vi "Maximum Corr coeff.vi"() -> (5 "Plug in titles":string[](array[string]), 7 "Plug in values":string[](array[string]))   [LabVIEW 2012]
uses:
  <vilib>/Analysis/3filter.llb/Filter Passband Type.ctl
  Globals/Meas_global.vi
  <vilib>/Analysis/3filter.llb/Zero Phase Filter (Cascade, DBL).vi
  <vilib>/Analysis/NI_AALBase.lvlib
panel:
  in  "Wind turbine location":dbl=10000.0
  out "XY Graph 3":cluster{"Time (ms)":dbl[], "Eng Values":dbl[]}[](graph)
  out "?":i32
  in  "Invert values?":bool
  in  "Filter 2nd Instrument data?":bool
  in  "Freq Cutoff Inst 2":dbl=100.0
  in  "Freq Cutoff Inst 1":dbl=100.0
  in  "Filter 1st Instrument Data?":bool
  out "Time for max corr coeff":dbl
  out "Max corr coeff":dbl
  in  "Start point":dbl
  in  "Time step":dbl
  in  "Input own variables?":bool=TRUE
  out "Start point":dbl
  out "XY Graph 2":cluster{dbl[], dbl[]}(graph)
  out "Time step":dbl
  in  "Number of estimates":i32
  out "XY Graph":cluster{"Time (ms)":dbl[], "Eng Values":dbl[]}[](graph)
  in  "Instrumnt 2":i32=1
  in  "Instrument 1":i32
  # "Time lag"
  # "Correlation"
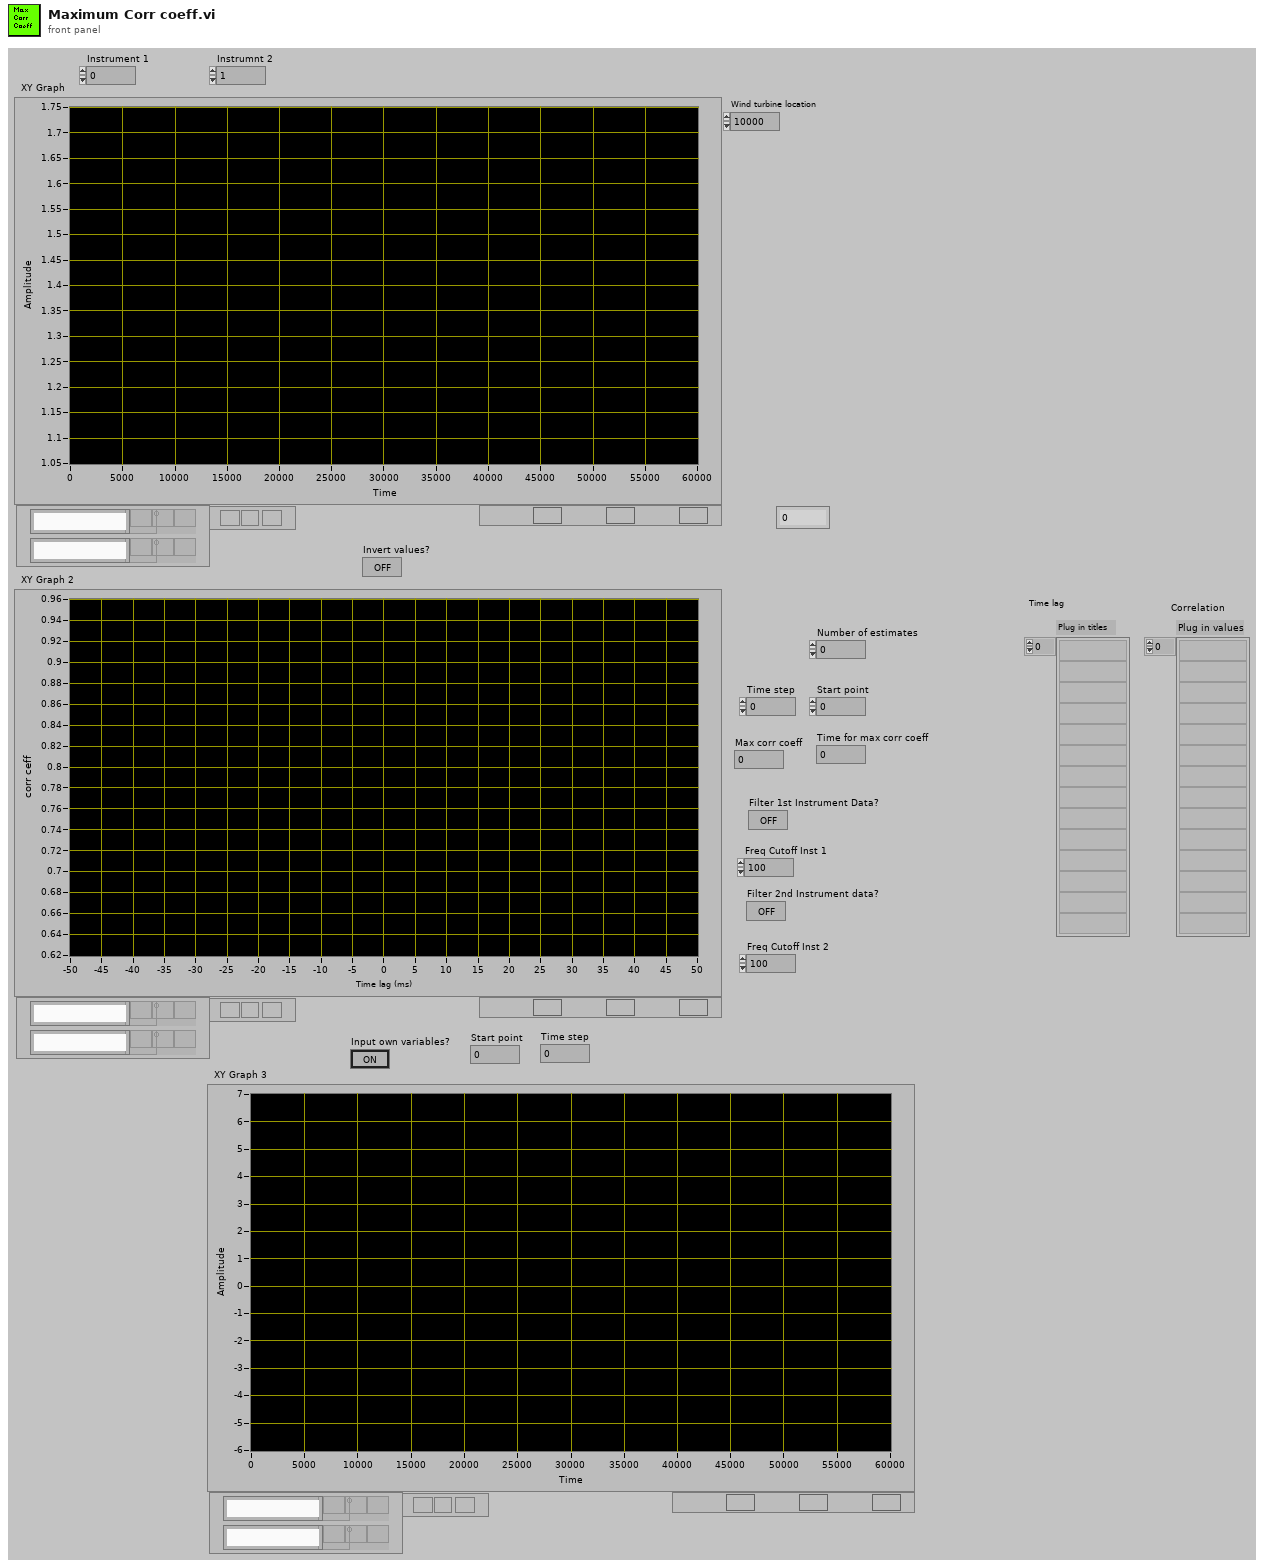
[diagram p1: front panel]
types:
  T1 = cluster{"Weighting":dbl[], "Time (ms)":dbl[], "Voltage":dbl[], "Eng Values":dbl[]}[]
  T2 = cluster{"Weighting":dbl[], "Time (ms)":dbl[], "Voltage":dbl[], "Eng Values":dbl[]}
  T3 = typedef "Analysis_info_cluster.ctl" = cluster{"Colour":u32, "Inst type":T4, "Inst name":string, "Symbol":string, "Code name":string, "Extra Info":string, "Inst Array":T5, "Extra Titles":string[], "Extra Values":string[], "U":dbl, "u^2":dbl, "u^3":dbl, "u^4":dbl, "Skew_u":dbl, "Kurt_u":dbl, "Sd Error in Mean":dbl, "% u'/U":dbl, "X":dbl, "Y":dbl, "Z":dbl, "Timescale integral to 25%":dbl, "Sd Error in Variance":dbl, "Calib File":path, "Calib Constants":dbl[], "Output Position":bool, "Full Stats":bool, "Av Sampling Rate":dbl, "Av No of Samples":dbl, "Total Meas Time (s)":dbl, "ADAM Ch Name":string}
  T4 = typedef "Inst_type.ctl" = enum16{"Propeller anemometer", "Raw voltage", "Pressure Transducer", "Pitot-static tube", "Preston tube", "Hot wire", "Cross wire 1", "Cross wire 2", "Generic Linear", "Generic Polynomial", "Generic BackPoly", "Fast FID", "Thermocouple", "Cold wire", "Pulsed Wire", "LDA Vel", "LDA Tran time", "LDA Arr time"}
  T5 = typedef "Instrument_Array.ctl" = enum16{"PWA", "LDA", "Analogue"}
  T6 = typedef "NI_AALBase.lvlib/Filter Passband Type.ctl" = enum32{"Lowpass", "Highpass", "Bandpass", "Bandstop"}
  T7 = cluster{"filter structure":enum32{"IIR 2nd Order", "IIR 4th Order"}, "Reverse Coefficients":dbl[], "Forward Coefficients":dbl[]}
  T8 = typedef "Correlation_cluster1.ctl" = cluster{"U inst":string, "uw":dbl, "u^2w":dbl, "uw^2":dbl, "uw/u'w'":dbl, "W inst":string, "uw^3":dbl, "u^3w":dbl, "u^2w^2":dbl, "Index U":i32, "Index W":i32}
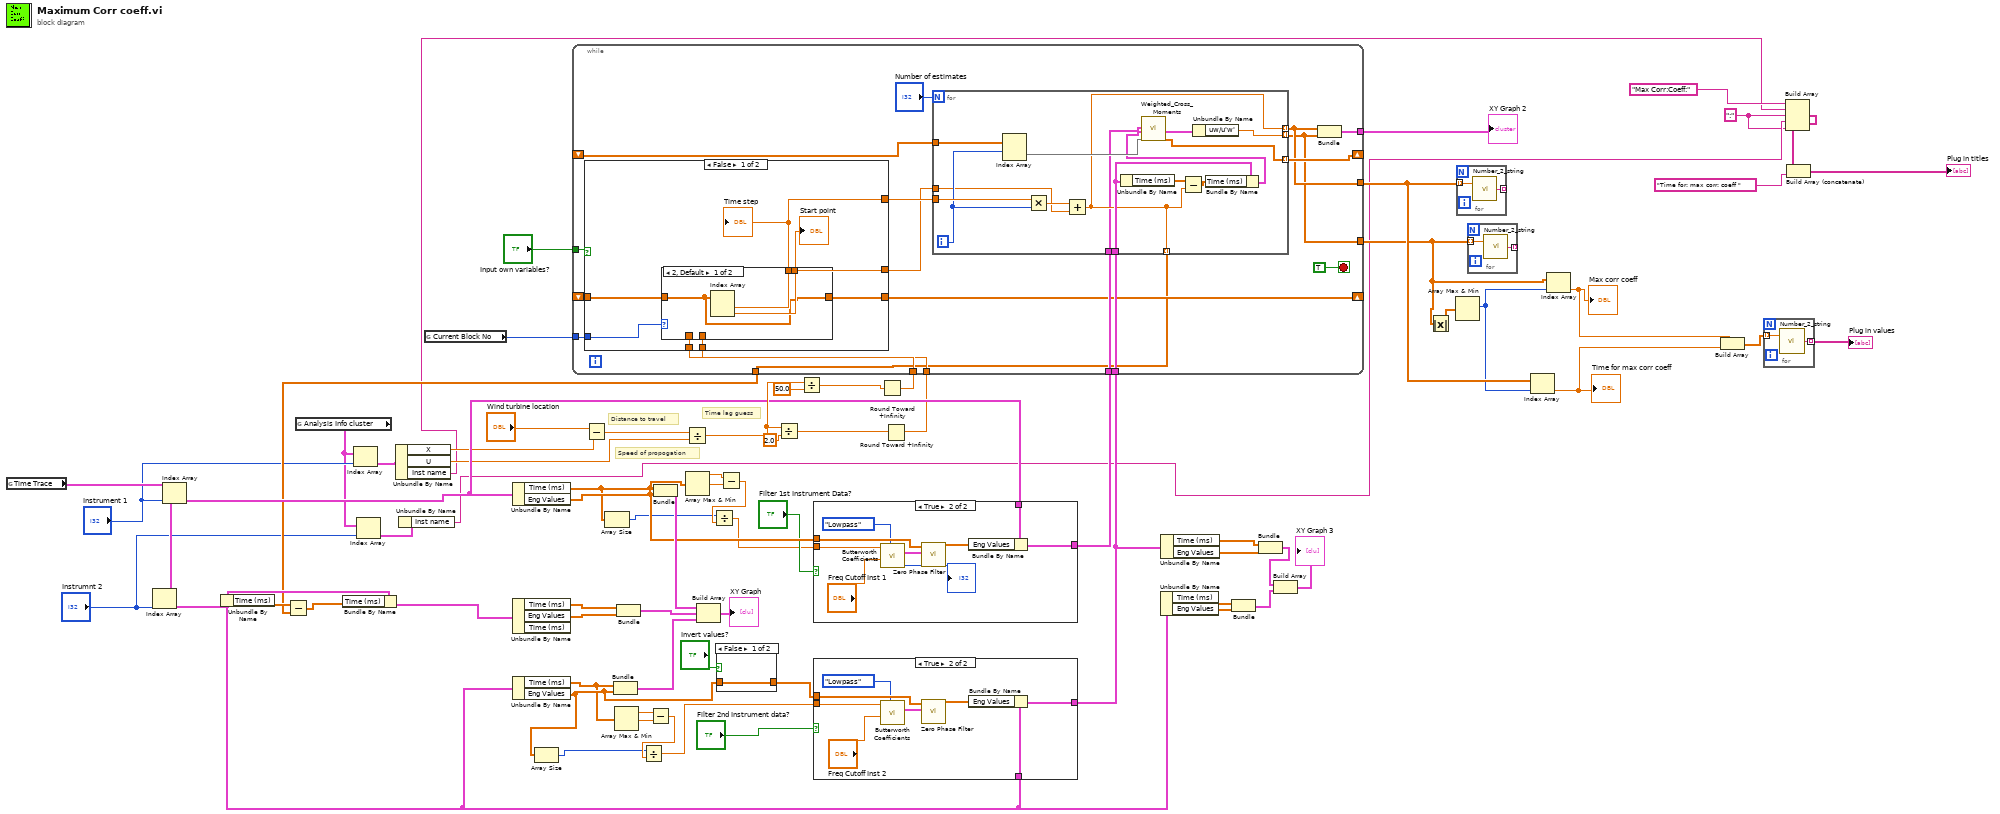
[diagram p0: block diagram]
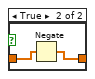
[diagram p2: hidden frame]
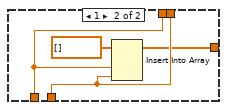
[diagram p5: hidden frame]
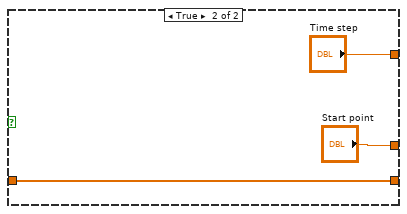
[diagram p6: hidden frame]
diagram:
  w1 = ":" ("element")
  # "Speed of propogation"
  # "Distance to travel"
  # "Time lag guess"
  n1 = global read "Meas_global.vi" "Time Trace"() -> (w68:T1)
  n2 = Index Array(array=w68, index="Instrumnt 2") -> (element=w43:T2)
  n3 = Index Array(array=w68, index="Instrument 1") -> (element=w45:T2)
  n4 = Unbundle By Name(w43) -> ("Time (ms)"=w67:dbl[])
  n5 = global read "Meas_global.vi" "Analysis Info cluster"() -> (w8:T3[])
  n6 = Index Array(array=w8, index="Instrument 1") -> (element=w22:T3)
  n7 = Index Array(array=w8, index="Instrumnt 2") -> (element=w9:T3)
  n8 = Unbundle By Name(w22) -> ("X"=w21:dbl, "U"=w20:dbl, "Inst name"=w5:string)
  n9 = Unbundle By Name(w9) -> ("Inst name"=w2:string)
  n10 = global read "Meas_global.vi" "Current Block No"() -> (w61:i32)
  n11 = Unbundle By Name(w45) -> ("Time (ms)"=w37:dbl[], "Eng Values"=w58:dbl[])
  n12 = Unbundle By Name(w43) -> ("Time (ms)"=w25:dbl[], "Eng Values"=w26:dbl[])
  n13 = Array Size(array=w26) -> (size(s)=w27:i32)
  n14 = Subtract(x="Wind turbine location", y=w21) -> (x-y=w19:dbl)
  n15 = Array Size(array=w37) -> (size(s)=w33:i32)
  n16 = Bundle("Time (ms)"=w25, "Eng Values"=w26) -> (w72:cluster{"Time (ms)":dbl[], "Eng Values":dbl[]})  [unwired: 1 in]
  n17 = Array Max & Min(array=w25) -> (max value=w29:dbl, min value=w30:dbl)  [unwired: 2 out]
  n18 = Subtract(x=w29, y=w30) -> (x-y=w28:dbl)
  n19 = Divide(x=w27, y=w28) -> (x/y=w31:dbl)
  n20 = Bundle("Time (ms)"=w37, "Eng Values"=w58) -> (w73:cluster{"Time (ms)":dbl[], "Eng Values":dbl[]})  [unwired: 1 in]
  n21 = Divide(x=w19, y=w20) -> (x/y=w63:dbl)
  n22 = Array Max & Min(array=w37) -> (max value=w36:dbl, min value=w35:dbl)  [unwired: 2 out]
  n23 = case shown="False" "Invert values?" {
    tunnel: w26 -> [w75 w76]
    tunnel: [w75 w77] -> w47
    frame False {
    }
    frame True {
      n24 = Negate(x=w76) -> (-x=w77:dbl[])
    }
  }
  n25 = Subtract(x=w36, y=w35) -> (x-y=w34:dbl)
  n26 = Divide(x=w33, y=w34) -> (x/y=w32:dbl)
  n27 = Divide(x=w63, y=2.0) -> (x/y=w17:dbl)
  n28 = Divide(x=w63, y=50.0) -> (x/y=w16:dbl)
  n29 = case shown="True" "Filter 1st Instrument Data?" {
    tunnel: w58 -> [_ w86]
    tunnel: w32 -> [_ w85]
    tunnel: w45 -> [w78 w83]
    tunnel: [w78 w82] -> w57
    frame False {
    }
    frame True {
      n30 = call <vilib>:"Butterworth Coefficients.vi"("filter type"=Filter_Passband_Type."Lowpass", "low cutoff freq: fl"="Freq Cutoff Inst 1", "sampling freq: fs"=w85) -> ("error"=→"?":i32, "IIR Filter Cluster"=w87:T7)  [unwired: 7 in]
      n31 = call-poly <vilib>:"Zero Phase Filter.vi"("IIR Filter Cluster"=w87, "X"=w86) -> ("Filtered X"=w84:dbl[])  [unwired: 8 in, 1 out]
      n32 = Bundle By Name(cluster=w83, "Eng Values"=w84) -> (w82:T2)
    }
  }
  n33 = case shown="True" "Filter 2nd Instrument data?" {
    tunnel: w47 -> [_ w95]
    tunnel: w31 -> [_ w94]
    tunnel: [w88 w92] -> w44
    tunnel: w43 -> [w88 w90]
    frame False {
    }
    frame True {
      n34 = call <vilib>:"Butterworth Coefficients.vi"("filter type"=Filter_Passband_Type."Lowpass", "low cutoff freq: fl"="Freq Cutoff Inst 2", "sampling freq: fs"=w94) -> ("IIR Filter Cluster"=w96:T7)  [unwired: 7 in, 1 out]
      n35 = call-poly <vilib>:"Zero Phase Filter.vi"("IIR Filter Cluster"=w96, "X"=w95) -> ("Filtered X"=w93:dbl[])  [unwired: 8 in, 1 out]
      n36 = Bundle By Name(cluster=w90, "Eng Values"=w93) -> (w92:T2)
    }
  }
  n37 = Round Toward +Infinity(x=w16) -> (ceil(x): smallest int >= x=w15:dbl)
  n38 = Round Toward +Infinity(x=w17) -> (ceil(x): smallest int >= x=w18:dbl)
  n39 = while {
    tunnel: w57 -> [w114]
    tunnel: w44 -> [w113]
    shift-right: [w111] -> _
    shift-left: _ -> [w110]
    tunnel: [w109] -> w65
    tunnel: [w107] -> w59
    tunnel: [w100] -> w38
    tunnel: w15 -> [w105]
    tunnel: w61 -> [w106]
    tunnel: w18 -> [w104]
    shift-right: [w103] -> _
    shift-left: _ -> [w102]
    tunnel: "Input own variables?" -> [w99]
    tunnel: [w97] -> w40
    stop <- TRUE stop-if-true
    n40 = case shown="False" w99 {
      tunnel: w106 -> [w121 _]
      tunnel: w105 -> [w120 _]
      tunnel: w104 -> [w119 _]
      tunnel: [w118 w129] -> w103
      tunnel: w102 -> [w117 w129]
      tunnel: [w116 "Start point"] -> w98
      tunnel: [w115 "Time step"] -> w101
      frame False {
        n41 = case shown="2, Default" w121 {
          tunnel: w120 -> [_ w127]
          tunnel: [w124 w127] -> w115
          tunnel: [w123 w128] -> w116
          tunnel: w119 -> [_ w128]
          tunnel: [w122 w126] -> w118
          tunnel: w117 -> [w122 _]
          frame 2, Default {
            n42 = Index Array(array=w122) -> (element #1=w124:dbl, element #2=w123:dbl)  [unwired: 2 in]
          }
          frame 1 {
            n43 = Insert Into Array(array=dbl[] [], new element #1=w127, new element #2=w128) -> (w126:dbl[])  [unwired: 1 in]
          }
        }
        "Time step" <- w115
        "Start point" <- w116
      }
      frame True {
      }
    }
    n44 = for {
      N: "Number of estimates" -> [_]
      tunnel: w114 -> [w133]
      tunnel: w113 -> [w138]
      tunnel: w101 -> [w146]
      tunnel: [w144] -> w111 mode=indexing
      tunnel: w110 -> [w143]
      tunnel: [w134] -> w107 mode=indexing
      tunnel: [w141] -> w100 mode=indexing
      tunnel: w98 -> [w135]
      tunnel: [w134] -> w97 mode=indexing
      i -> [w137]
      n45 = Index Array(array=w143, index (row)=w137) -> (element=w145:dbl[])  [unwired: 1 in]
      n46 = Multiply(x=w146, y=w137) -> (x*y=w136:dbl)
      n47 = Add(x=w136, y=w135) -> (x+y=w134:dbl)
      n48 = Unbundle By Name(w138) -> ("Time (ms)"=w140:dbl[])
      n49 = Subtract(x=w140, y=w134) -> (x-y=w139:dbl[])
      n50 = Bundle By Name(cluster=w138, "Time (ms)"=w139) -> (w132:T2)
      n51 = call "Weighted_Cross_Moments.vi"("Time Cluster 1"=w133, "Time Cluster 2"=w132, "Shift in"=w145) -> ("output cluster"=w142:T8, "Shift out"=w144:dbl[])  [unwired: 15 in]
      n52 = Unbundle By Name(w142) -> ("uw/u'w'"=w141:dbl)
    }
    n53 = Bundle(w107, w100) -> (w109:cluster{dbl[], dbl[]})  [unwired: 1 in]
  }
  "XY Graph 2" <- w65
  n54 = Subtract(x=w67, y=w40) -> (x-y=w66:dbl[])
  n55 = Bundle By Name(cluster=w43, "Time (ms)"=w66) -> (w46:T2)
  n56 = Unbundle By Name(w46) -> ("Time (ms)"=w70:dbl[], "Eng Values"=w69:dbl[])  [unwired: 1 out]
  n57 = Bundle("Time (ms)"=w70, "Eng Values"=w69) -> (w74:cluster{"Time (ms)":dbl[], "Eng Values":dbl[]})  [unwired: 1 in]
  n58 = Build Array(w73, w74, w72) -> (→"XY Graph":cluster{"Time (ms)":dbl[], "Eng Values":dbl[]}[])
  n59 = Unbundle By Name(w43) -> ("Time (ms)"=w50:dbl[], "Eng Values"=w49:dbl[])
  n60 = Unbundle By Name(w44) -> ("Time (ms)"=w52:dbl[], "Eng Values"=w51:dbl[])
  n61 = Bundle("Time (ms)"=w50, "Eng Values"=w49) -> (w42:cluster{"Time (ms)":dbl[], "Eng Values":dbl[]})  [unwired: 1 in]
  n62 = Bundle("Time (ms)"=w52, "Eng Values"=w51) -> (w41:cluster{"Time (ms)":dbl[], "Eng Values":dbl[]})  [unwired: 1 in]
  n63 = Build Array(w41, w42) -> (→"XY Graph 3":cluster{"Time (ms)":dbl[], "Eng Values":dbl[]}[])
  n64 = Absolute Value(x=w38) -> (abs(x)=w54:dbl[])
  n65 = Array Max & Min(array=w54) -> (max index (indices)=w39:i32)  [unwired: 3 out]
  n66 = for {
    tunnel: w59 -> [w147] mode=indexing
    tunnel: [w148] -> _ mode=indexing
    n67 = call "Number_2_string.vi"("number"=w147) -> ("String"=w148:string)  [unwired: 1 in]
  }
  n68 = for {
    tunnel: w38 -> [w149] mode=indexing
    tunnel: [w150] -> _ mode=indexing
    n69 = call "Number_2_string.vi"("number"=w149) -> ("String"=w150:string)  [unwired: 1 in]
  }
  n70 = Index Array(array=w59, index=w39) -> (element=w11:dbl)
  "Time for max corr coeff" <- w11
  n71 = Index Array(array=w38, index=w39) -> (element=w12:dbl)
  "Max corr coeff" <- w12
  n72 = Build Array(w12, w11) -> (w14:dbl[])
  n73 = for {
    tunnel: w14 -> [w151] mode=indexing
    tunnel: [w152] -> w13 mode=indexing
    n74 = call "Number_2_string.vi"("number"=w151) -> ("String"=w152:string)  [unwired: 1 in]
  }
  "Plug in values" <- w13
  n75 = Build Array("Max Corr:Coeff:", w5, w1, w2, w1) -> (w3:string[])
  n76 = Build Array (concatenate)(w3, "Time for: max corr: coeff ") -> (→"Plug in titles":string[])
